vi "deposit.vi"(1 "Elements+Rates":cluster{"Elements":u16[], "Rates":sgl[]}, 2 "# of units":i32, 3 "Input array":T2(array[cluster])) -> (0 "Deposit again?":bool)   [LabVIEW 2012]
uses:
  elements.gbl
  active_process.gbl
  shutter_timeout.gbl
  number_of_sources.gbl
panel:
  in  "Rates":T1
  out "Repeating unit #":i32
  out "Display":string
  in  "Emergency":bool
  in  "Abort":bool
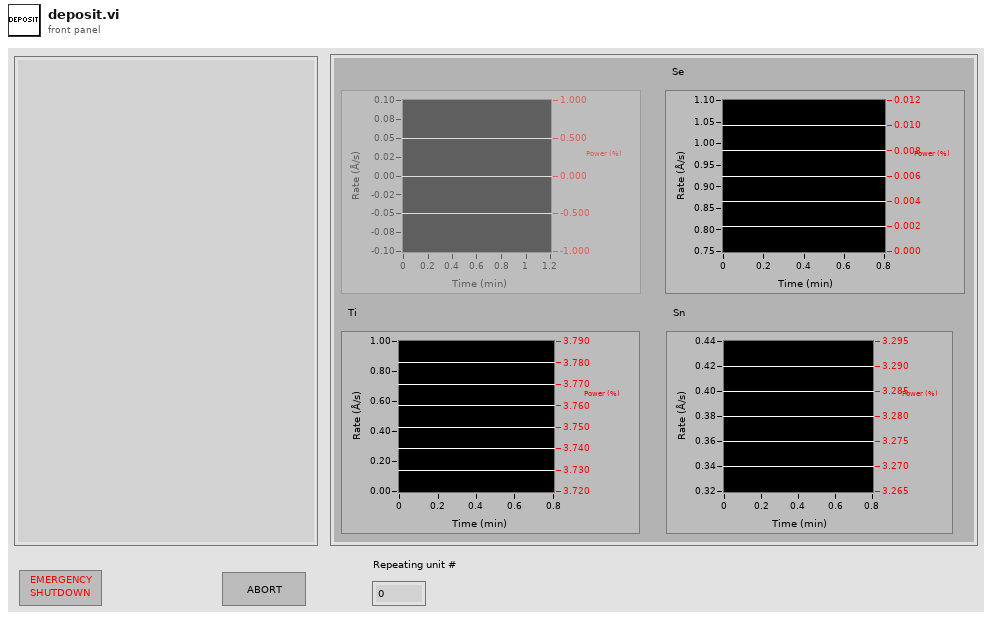
[diagram p1: front panel]
types:
  T1 = cluster{"Rate graph":cluster{cluster{sgl, "Numeric":sgl}[]}[], "Rate graph 2":cluster{cluster{sgl, "Numeric":sgl}[]}[], "Rate graph 3":cluster{cluster{sgl, "Numeric":sgl}[]}[], "Rate graph 4":cluster{cluster{sgl, "Numeric":sgl}[]}[]}
  T2 = cluster{"Elements":u8[][], "T|D":bool[], "T (Å) / D (s)":sgl[], "Repeats":i32}[]
  T3 = enum8{"Enabled", "Disabled", "Disabled and Grayed Out"}
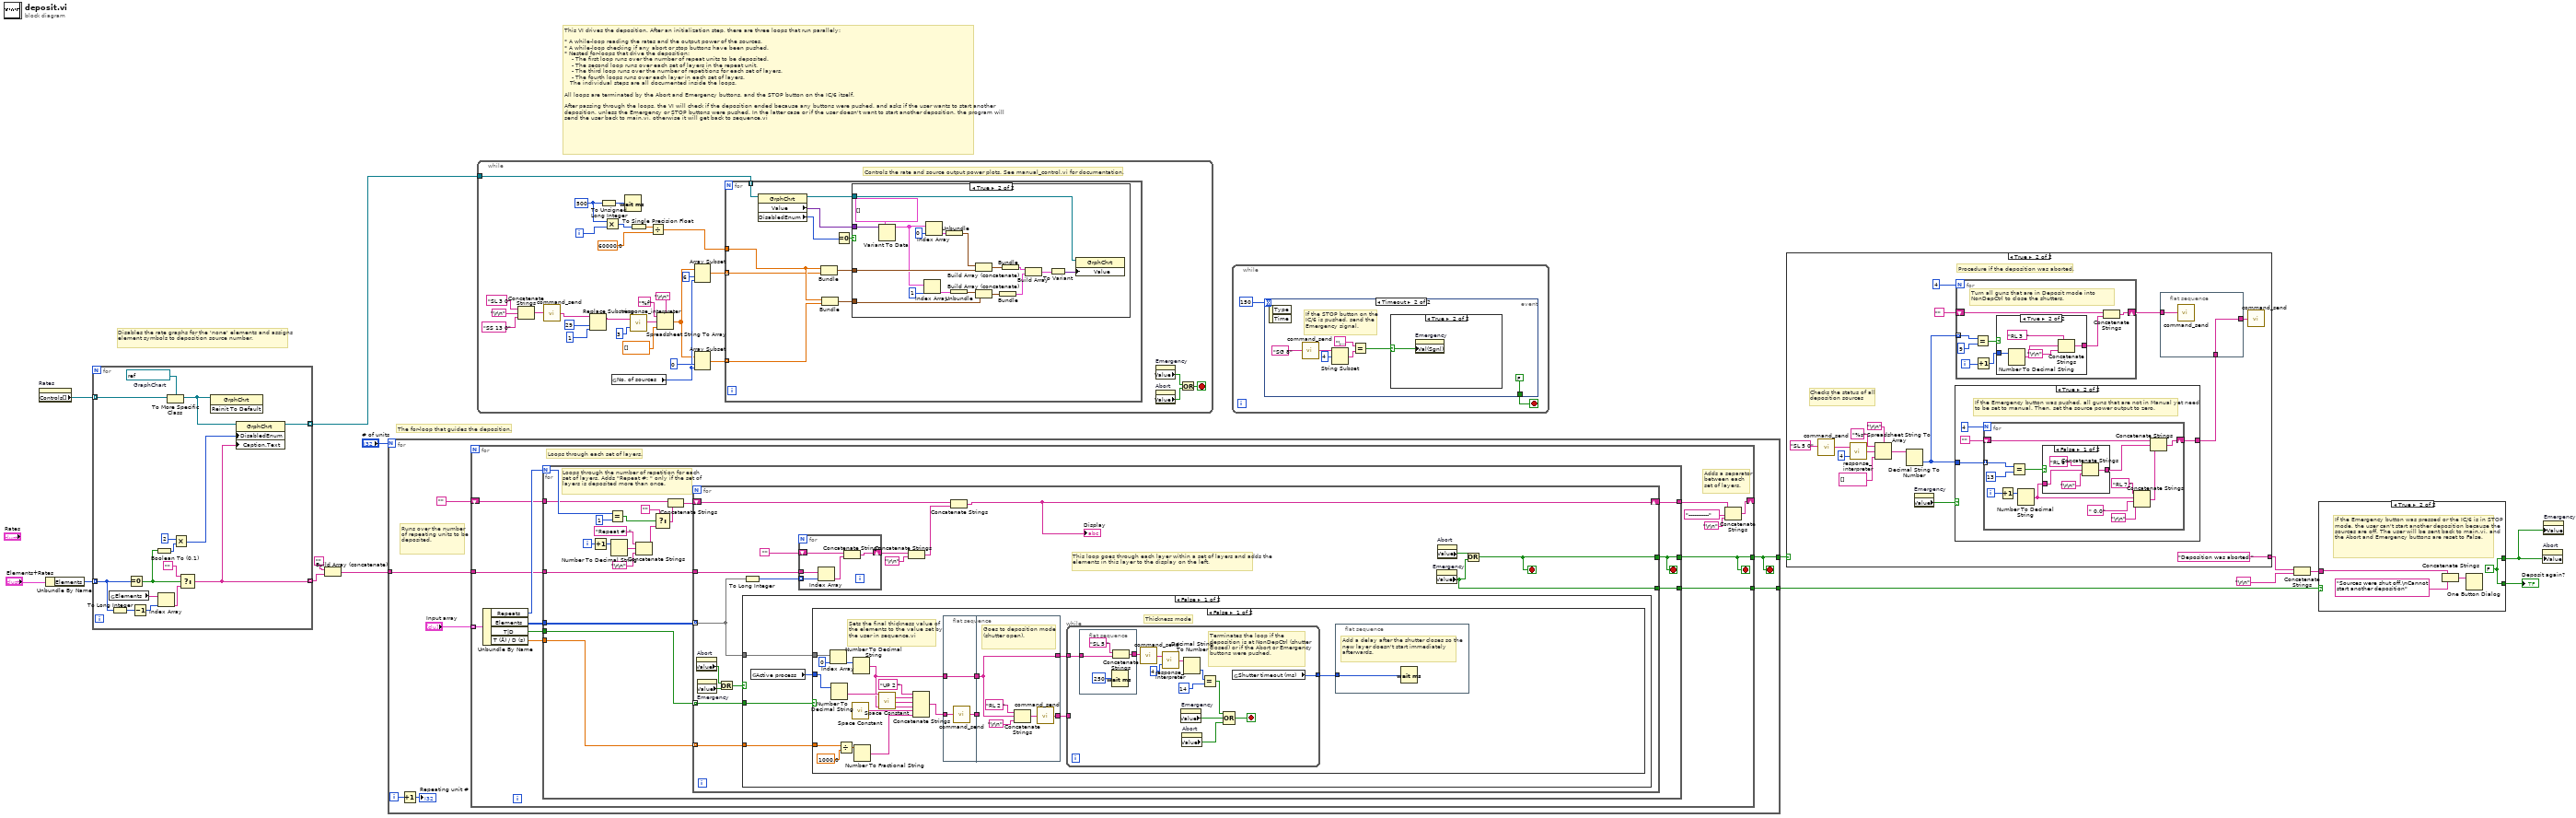
[diagram p0: block diagram]
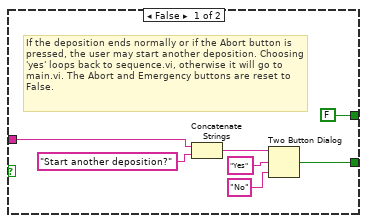
[diagram p2: hidden frame]
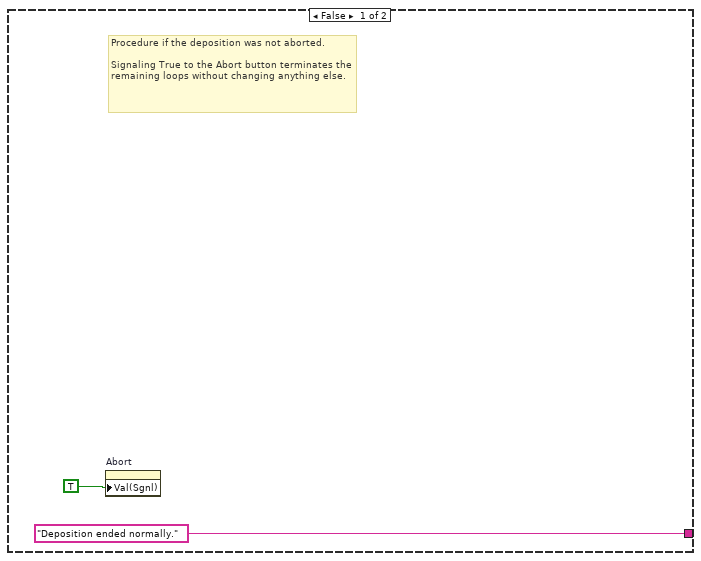
[diagram p3: hidden frame]
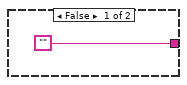
[diagram p4: hidden frame]
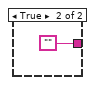
[diagram p5: hidden frame]
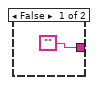
[diagram p6: hidden frame]
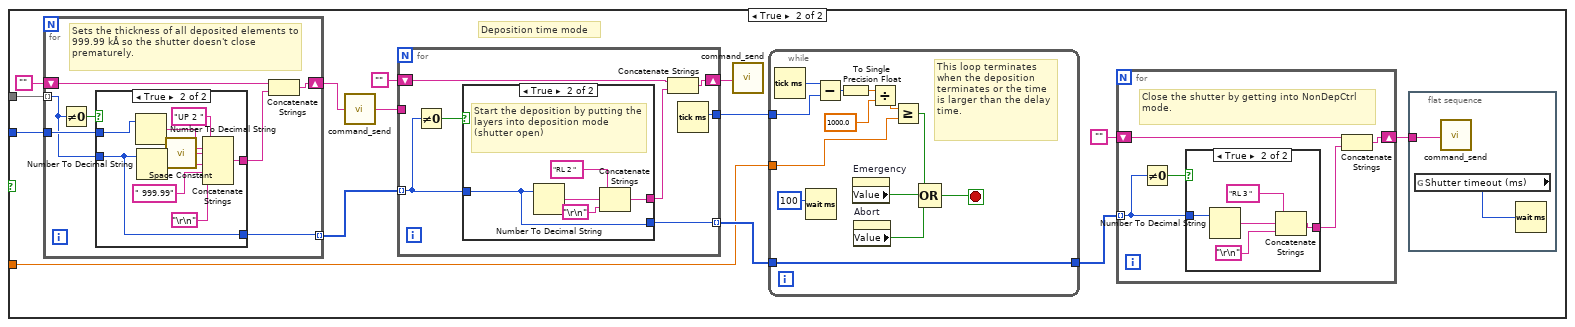
[diagram p7: hidden frame]
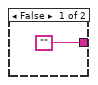
[diagram p8: hidden frame]
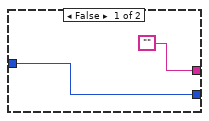
[diagram p9: hidden frame]
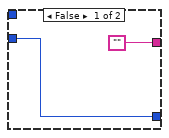
[diagram p10: hidden frame]
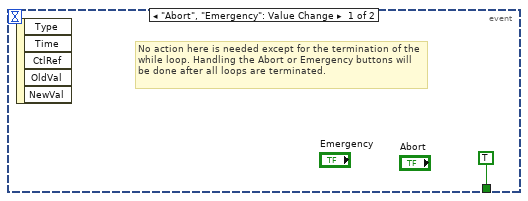
[diagram p13: hidden frame]
diagram:
  # "The for-loop that guides the deposition."
  # "Disables the rate graphs for the 'none' elements and assigns element symbols to deposition source number."
  # "This VI drives the deposition. After an initialization step, there are three loops that run parallely:\n\n* A while-loop reading the rates and the output power of the sources.\n* A while-loop checking if any abort or stop buttons have been pushed. \n* Nested for-loops that drive the deposition:\n    - The first loop runs over the number of repeat units to be deposited.\n    - The second loop runs over each set of layers in the repeat unit.\n    - The third loop runs over the number of repetitions for each set of layers.\n    - The fourth loops runs over each layer in each set of layers.\n   The individual steps are all documented inside the loops.\n\nAll loops are terminated by the Abort and Emergency buttons, and the STOP button on the IC/6 itself.\n\nAfter passing through the loops, the VI will check if the deposition ended because any buttons were pushed, and asks if the user wants to start another deposition, unless the Emergency or STOP buttons were pushed. In the latter case or if the user doesn't want to start another deposition, the program will send the user back to main.vi, otherwise it will get back to sequence.vi"
  n1 = property on="Rates" class="Clust (strict)"() -> ("Controls[]"=w2:refnum<vi>[])  [unwired: 2 in, 2 out]
  n2 = Unbundle By Name("Elements+Rates") -> ("Elements"=w14:u16[])
  n3 = for {
    tunnel: w14 -> [w26] mode=indexing
    tunnel: [w19] -> w8 mode=indexing
    tunnel: w2 -> [w21] mode=indexing
    tunnel: [w17] -> w1 mode=indexing
    w22 = refnum<vi> refnum  # GraphChart
    n4 = global read "elements.gbl" "Elements"() -> (w30:string[])
    n5 = To Long Integer(number=w26) -> (32bit integer=w16:i32)
    n6 = Equal To 0?(x=w26) -> (x = 0?=w23:bool)
    n7 = Decrement(x=w16) -> (x-1=w29:i32)
    n8 = Boolean To (0,1)(Boolean=w23) -> (0, 1=w27:i16)
    n9 = Index Array(array=w30, index=w29) -> (element=w25:string)
    n10 = To More Specific Class(target class=w22, reference=w21) -> (specific class reference=w20:refnum<vi>)  [unwired: 1 in, 1 out]
    n11 = Multiply(x=i16 2, y=w27) -> (x*y=w18:i16)
    n12 = Select(t="", s=w23, f=w25) -> (s? t:f=w19:string)
    n13 = invoke class="GrphChrt" method="Reinit To Default"(reference=w20) -> ()  [unwired: 2 in, 3 out]
    n14 = property class="GrphChrt"(reference=w20, "DisabledEnum"=w18, "Caption.Text"=w19) -> (reference out=w17:refnum<vi>)  [unwired: 1 in, 1 out]
  }
  n15 = Build Array (concatenate)("", w8) -> (w5:string[])
  n16 = for {
    N: "# of units" -> [_]
    tunnel: w5 -> [w34]
    tunnel: [w33] -> w9
    tunnel: [w32] -> w6
    i -> [w36]
    stop <- w33 stop-if-true
    # "Runs over the number of repeating units to be deposited."
    n17 = Increment(x=w36) -> (x+1=→"Repeating unit #":i32)
    n18 = for {
      tunnel: w34 -> [w41]
      shift-right: [w47] -> _
      shift-left: "" -> [w40]
      tunnel: [w46] -> w33
      tunnel: [w45] -> w32
      tunnel: "Input array" -> [w44] mode=indexing
      stop <- w46 stop-if-true
      # "Loops through each set of layers."
      # "Adds a separator between each set of layers."
      n19 = Unbundle By Name(w44) -> ("Repeats"=w43:i32, "Elements"=w42:u8[][], "T|D"=w39:bool[], "T (Å) / D (s)"=w38:sgl[])
      n20 = for {
        N: w43 -> [w57]
        tunnel: w40 -> [w54]
        tunnel: w41 -> [w70]
        tunnel: [w69] -> w48
        tunnel: [w56] -> w46
        tunnel: [w55] -> w45
        tunnel: w42 -> [w53]
        tunnel: w39 -> [w52]
        tunnel: w38 -> [w51]
        i -> [w63]
        stop <- w56 stop-if-true
        # "Loops through the number of repetition for each set of layers. Adds \"Repeat #: \" only if the set of layers is deposited more than once."
        n21 = Increment(x=w63) -> (x+1=w67:i32)
        n22 = Equal?(x=w57, y=1) -> (x = y?=w59:bool)
        n23 = Number To Decimal String(number=w67) -> (decimal integer string=w66:string)  [unwired: 1 in]
        n24 = Concatenate Strings("Repeat #: ", w66, "\r\n") -> (w62:string)
        n25 = Select(t="", s=w59, f=w62) -> (s? t:f=w61:string)
        n26 = Concatenate Strings(w54, w61) -> (w68:string)
        n27 = for {
          tunnel: w53 -> [w85] mode=indexing
          tunnel: w52 -> [w87] mode=indexing
          tunnel: w51 -> [w86] mode=indexing
          shift-right: [w78] -> w69
          shift-left: w68 -> [w80]
          tunnel: w70 -> [w84]
          tunnel: [w75] -> w56
          tunnel: [w76] -> w55
          stop <- w75 stop-if-true
          # "This loop goes through each layer within a set of layers and adds the elements in this layer to the display on the left."
          n28 = property on="Abort" class="Bool (strict)"() -> ("Value"=w72:bool)  [unwired: 2 in, 2 out]
          n29 = property on="Emergency" class="Bool (strict)"() -> ("Value"=w73:bool)  [unwired: 2 in, 2 out]
          n30 = Or(x=w72, y=w73) -> (x .or. y?=w74:bool)
          n31 = case shown="False" w74 {
            tunnel: w87 -> [w91 _]
            tunnel: w86 -> [w90 _]
            tunnel: w85 -> [w89 _]
            frame False {
              n32 = global read "active_process.gbl" "Active process"() -> (w88:i32)
              n33 = case shown="False" w91 {
                tunnel: w90 -> [w107 w141]
                tunnel: w89 -> [w98 w149]
                tunnel: w88 -> [w92 w136]
                frame False {
                  # "Sets the final thickness value of the elements to the value set by the user in sequence.vi"
                  # "Thickness mode"
                  n34 = Index Array(array=w98, index=0) -> (element=w109:u8)
                  n35 = Number To Decimal String(number=w92) -> (decimal integer string=w94:string)  [unwired: 1 in]
                  n36 = Divide(x=w107, y=sgl 1000.0) -> (x/y=w105:sgl)
                  n37 = call <vilib>:"Space Constant.vi"() -> ("String"=w108:string)
                  n38 = Number To Decimal String(number=w109) -> (decimal integer string=w93:string)  [unwired: 1 in]
                  n39 = Number To Fractional String(number=w105) -> (F-format string=w104:string)  [unwired: 3 in]
                  n40 = call <vilib>:"Space Constant.vi"() -> ("String"=w95:string)
                  n41 = Concatenate Strings("UP 2 ", w94, w95, w93, w108, w104) -> (w103:string)
                  n42 = flat-sequence {
                    tunnel: w103 -> [w130]
                    tunnel: w93 -> [w129]
                    tunnel: [w129] -> w102
                    tunnel: [w128] -> w97
                    tunnel: w102 -> [w132]
                    tunnel: [w132] -> w100
                    tunnel: [w131] -> w99
                    tunnel: w97 -> [_]
                    frame #0 {
                      n43 = call "command_send.vi"("Commands"=w130) -> ("Response"=w128:string)
                    }
                    frame #1 {
                      # "Goes to deposition mode (shutter open)."
                      n44 = Concatenate Strings("RL 2 ", w132, "\r\n") -> (w133:string)
                      n45 = call "command_send.vi"("Commands"=w133) -> ("Response"=w131:string)
                    }
                  }
                  n46 = while {
                    tunnel: [w111] -> w101
                    tunnel: w100 -> [w112]
                    tunnel: w99 -> [_]
                    stop <- w113 stop-if-true
                    # "Terminates the loop if the deposition is at NonDepCtrl (shutter closed) or if the Abort or Emergency buttons were pushed."
                    n47 = flat-sequence {
                      tunnel: [w125] -> w120
                      tunnel: w112 -> [w124]
                      frame #0 {
                        n48 = Wait (ms)(milliseconds to wait=u32 250) -> ()  [unwired: 1 out]
                        n49 = Concatenate Strings("SL 5 ", w124) -> (w125:string)
                      }
                    }
                    n50 = call "command_send.vi"("Commands"=w120) -> ("Response"=w119:string)
                    n51 = call "response_interpreter.vi"("Response type"=u16 4, "Response hex"=w119) -> ("Response (readable)"=w116:string)
                    n52 = property on="Emergency" class="Bool (strict)"() -> ("Value"=w121:bool)  [unwired: 2 in, 2 out]
                    n53 = property on="Abort" class="Bool (strict)"() -> ("Value"=w122:bool)  [unwired: 2 in, 2 out]
                    n54 = Decimal String To Number(string=w116) -> (number=w115:i32)  [unwired: 2 in, 1 out]
                    n55 = Equal?(x=w115, y=14) -> (x = y?=w114:bool)
                    n56 = Compound Arithmetic op=OR(w114, w121, w122) -> (w113:bool)
                    n57 = global read "shutter_timeout.gbl" "Shutter timeout (ms)"() -> (w111:u32)
                  }
                  n58 = flat-sequence {
                    tunnel: w101 -> [w127]
                    frame #0 {
                      # "Add a delay after the shutter closes so the new layer doesn't start immediately afterwards."
                      n59 = Wait (ms)(milliseconds to wait=w127) -> ()  [unwired: 1 out]
                    }
                  }
                }
                frame True {
                  # "Deposition time mode"
                  n60 = for {
                    tunnel: w149 -> [w190] mode=indexing
                    shift-right: [w193] -> w147
                    shift-left: "" -> [w195]
                    tunnel: [w192] -> w146 mode=indexing
                    tunnel: w136 -> [w191]
                    # "Sets the thickness of all deposited elements to 999.99 kÅ so the shutter doesn't close prematurely."
                    n61 = Not Equal To 0?(x=w190) -> (x != 0?=w196:bool)
                    n62 = case shown="True" w196 {
                      tunnel: w190 -> [w197 w203]
                      tunnel: ["" w204] -> w194
                      tunnel: [w197 w203] -> w192
                      tunnel: w191 -> [_ w199]
                      frame False {
                      }
                      frame True {
                        n63 = Number To Decimal String(number=w199) -> (decimal integer string=w200:string)  [unwired: 1 in]
                        n64 = Number To Decimal String(number=w203) -> (decimal integer string=w206:string)  [unwired: 1 in]
                        n65 = call <vilib>:"Space Constant.vi"() -> ("String"=w202:string)
                        n66 = Concatenate Strings("UP 2 ", w200, w202, w206, " 999.99", "\r\n") -> (w204:string)
                      }
                    }
                    n67 = Concatenate Strings(w195, w194) -> (w193:string)
                  }
                  n68 = call "command_send.vi"("Commands"=w147) -> ("Response"=w137:string)
                  n69 = for {
                    tunnel: w146 -> [w181] mode=indexing
                    shift-right: [w178] -> w144
                    shift-left: "" -> [w180]
                    tunnel: [w177] -> w142 mode=indexing
                    tunnel: [w176] -> w143
                    tunnel: w137 -> [_]
                    n70 = Not Equal To 0?(x=w181) -> (x != 0?=w182:bool)
                    n71 = case shown="True" w182 {
                      tunnel: w181 -> [w183 w186]
                      tunnel: ["" w187] -> w179
                      tunnel: [w183 w186] -> w177
                      frame False {
                      }
                      frame True {
                        # "Start the deposition by putting the layers into deposition mode (shutter open)"
                        n72 = Number To Decimal String(number=w186) -> (decimal integer string=w189:string)  [unwired: 1 in]
                        n73 = Concatenate Strings("RL 2 ", w189, "\r\n") -> (w187:string)
                      }
                    }
                    n74 = Concatenate Strings(w180, w179) -> (w178:string)
                    n75 = Tick Count (ms)() -> (millisecond timer value=w176:u32)
                  }
                  n76 = call "command_send.vi"("Commands"=w144) -> ()  [unwired: 1 out]
                  n77 = while {
                    tunnel: w143 -> [w174]
                    tunnel: w141 -> [w170]
                    tunnel: w142 -> [w164]
                    tunnel: [w164] -> w138
                    stop <- w165 stop-if-true
                    # "This loop terminates when the deposition terminates or the time is larger than the delay time."
                    n78 = Tick Count (ms)() -> (millisecond timer value=w175:u32)
                    n79 = Wait (ms)(milliseconds to wait=u32 100) -> ()  [unwired: 1 out]
                    n80 = Subtract(x=w175, y=w174) -> (x-y=w173:u32)
                    n81 = To Single Precision Float(number=w173) -> (single precision float=w163:sgl)
                    n82 = property on="Emergency" class="Bool (strict)"() -> ("Value"=w167:bool)  [unwired: 2 in, 2 out]
                    n83 = property on="Abort" class="Bool (strict)"() -> ("Value"=w168:bool)  [unwired: 2 in, 2 out]
                    n84 = Divide(x=w163, y=sgl 1000.0) -> (x/y=w171:sgl)
                    n85 = Greater Or Equal?(x=w171, y=w170) -> (x >= y?=w166:bool)
                    n86 = Compound Arithmetic op=OR(w166, w167, w168) -> (w165:bool)
                  }
                  n87 = for {
                    tunnel: w138 -> [w155] mode=indexing
                    shift-right: [w152] -> w140
                    shift-left: "" -> [w154]
                    # "Close the shutter by getting into NonDepCtrl mode."
                    n88 = Not Equal To 0?(x=w155) -> (x != 0?=w156:bool)
                    n89 = case shown="True" w156 {
                      tunnel: w155 -> [_ w159]
                      tunnel: ["" w160] -> w153
                      frame False {
                      }
                      frame True {
                        n90 = Number To Decimal String(number=w159) -> (decimal integer string=w162:string)  [unwired: 1 in]
                        n91 = Concatenate Strings("RL 3 ", w162, "\r\n") -> (w160:string)
                      }
                    }
                    n92 = Concatenate Strings(w154, w153) -> (w152:string)
                  }
                  n93 = flat-sequence {
                    tunnel: w140 -> [w151]
                    frame #0 {
                      n94 = global read "shutter_timeout.gbl" "Shutter timeout (ms)"() -> (w150:u32)
                      n95 = call "command_send.vi"("Commands"=w151) -> ()  [unwired: 1 out]
                      n96 = Wait (ms)(milliseconds to wait=w150) -> ()  [unwired: 1 out]
                    }
                  }
                }
              }
            }
            frame True {
              # "If this condition isn't set, the VI will start depositing the current layer even when it should abort the deposition."
            }
          }
          n97 = To Long Integer(number=w85) -> (32bit integer=w71:i32[])
          n98 = for {
            tunnel: w71 -> [w208] mode=indexing
            tunnel: w84 -> [w209]
            shift-right: [w211] -> w82
            shift-left: "" -> [w212]
            n99 = Index Array(array=w209, index=w208) -> (element=w210:string)
            n100 = Concatenate Strings(w212, w210) -> (w211:string)
          }
          n101 = Concatenate Strings(w82, "\r\n") -> (w79:string)
          n102 = Concatenate Strings(w80, w79) -> (w78:string)
          "Display" <- w78
          n103 = property on="Emergency" class="Bool (strict)"() -> ("Value"=w76:bool)  [unwired: 2 in, 2 out]
          n104 = property on="Abort" class="Bool (strict)"() -> ("Value"=w77:bool)  [unwired: 2 in, 2 out]
          n105 = Or(x=w77, y=w76) -> (x .or. y?=w75:bool)
        }
      }
      n106 = Concatenate Strings(w48, "-----------", "\r\n") -> (w47:string)
    }
  }
  n107 = while {
    tunnel: w1 -> [w234]
    i -> [w239]
    stop <- w240 stop-if-true
    w238 = 500
    # "Controls the rate and source output power plots. See manual_control.vi for documentation."
    n108 = Concatenate Strings("SL 3 0", "\r\n", "SS 13 0") -> (w225:string)
    n109 = call "command_send.vi"("Commands"=w225) -> ("Response"=w216:string)
    n110 = Replace Substring(2:1, 3:29, 5:w216) -> (1:w217:string)  [unwired: 1 in, 1 out]
    n111 = To Unsigned Long Integer(number=w238) -> (unsigned 32bit integer=w213:u32)
    n112 = Multiply(x=w238, y=w239) -> (x*y=w237:i32)
    n113 = global read "number_of_sources.gbl" "No. of sources"() -> (w220:i32)
    n114 = Wait (ms)(milliseconds to wait=w213) -> ()  [unwired: 1 out]
    n115 = call "response_interpreter.vi"("Response type"=u16 3, "Response hex"=w217) -> ("Response (readable)"=w230:string)
    n116 = To Single Precision Float(number=w237) -> (single precision float=w218:sgl)
    n117 = Divide(x=w218, y=sgl 60000.0) -> (x/y=w235:sgl)
    n118 = Spreadsheet String To Array(delimiter (Tab)="\r\n", format string="%f", spreadsheet string=w230, array type (2D Dbl)=sgl[] []) -> (array=w219:sgl[])
    n119 = Array Subset(array=w219, index=6, length=w220) -> (w224:sgl[])
    n120 = Array Subset(array=w219, index=0, length=w220) -> (w223:sgl[])
    n121 = for {
      tunnel: w224 -> [w248] mode=indexing
      tunnel: w235 -> [w252]
      tunnel: w223 -> [w247] mode=indexing
      tunnel: w234 -> [w246] mode=indexing
      n122 = property class="GrphChrt"(reference=w246) -> (reference out=w245:refnum<vi>, "Value"=w243:variant, "DisabledEnum"=w244:T3)  [unwired: 1 in, 1 out]
      n123 = Bundle(w252, w248) -> (w250:cluster{sgl, sgl})  [unwired: 1 in]
      n124 = Bundle(w252, w247) -> (w251:cluster{sgl, sgl})  [unwired: 1 in]
      n125 = Equal To 0?(x=w244) -> (x = 0?=w249:bool)
      n126 = case shown="True" w249 {
        tunnel: w251 -> [_ w266]
        tunnel: w250 -> [_ w262]
        tunnel: w243 -> [_ w254]
        tunnel: w245 -> [_ w257]
        frame False {
        }
        frame True {
          n127 = Variant To Data(type=cluster{cluster{sgl, sgl}[]}[] [], Variant=w254) -> (data=w255:cluster{cluster{sgl, sgl}[]}[])  [unwired: 1 in, 1 out]
          n128 = Index Array(array=w255, index=1) -> (element=w260:cluster{cluster{sgl, sgl}[]})
          n129 = Index Array(array=w255, index=0) -> (element=w263:cluster{cluster{sgl, sgl}[]})
          n130 = Unbundle(w263) -> (w261:cluster{sgl, sgl}[])
          n131 = Unbundle(w260) -> (w259:cluster{sgl, sgl}[])
          n132 = Build Array (concatenate)(w261, w262) -> (w269:cluster{sgl, sgl}[])
          n133 = Build Array (concatenate)(w259, w266) -> (w270:cluster{sgl, sgl}[])
          n134 = Bundle(w270) -> (w267:cluster{cluster{sgl, sgl}[]})  [unwired: 1 in]
          n135 = Bundle(w269) -> (w268:cluster{cluster{sgl, sgl}[]})  [unwired: 1 in]
          n136 = Build Array(w268, w267) -> (w258:cluster{cluster{sgl, sgl}[]}[])
          n137 = To Variant(anything=w258) -> (Variant=w256:variant)
          n138 = property class="GrphChrt"(reference=w257, "Value"=w256) -> ()  [unwired: 1 in, 2 out]
        }
      }
    }
    n139 = property on="Emergency" class="Bool (strict)"() -> ("Value"=w242:bool)  [unwired: 2 in, 2 out]
    n140 = property on="Abort" class="Bool (strict)"() -> ("Value"=w241:bool)  [unwired: 2 in, 2 out]
    n141 = Or(x=w242, y=w241) -> (x .or. y?=w240:bool)
  }
  n142 = while {
    stop <- w272 stop-if-true
    n143 = event shown="[1] Timeout" {
      selector: _ -> [_ _]
      dyn-events: _ -> [_ _]
      timeout: 150 -> [_ _]
      tunnel: [TRUE FALSE] -> w272
      event "Abort", "Emergency": Value Change {
        # "No action here is needed except for the termination of the while loop. Handling the Abort or Emergency buttons will be done after all loops are terminated."
        n144 = event-data() -> ()  [unwired: 1 in, 5 out]
      }
      event Timeout {
        # "If the STOP button on the IC/6 is pushed, send the Emergency signal."
        n145 = event-data() -> ()  [unwired: 1 in, 2 out]
        n146 = call "command_send.vi"("Commands"="SG 8") -> ("Response"=w279:string)
        n147 = String Subset(string=w279, offset (0)=4) -> (substring=w276:string)  [unwired: 1 in]
        n148 = Equal?(x="\u0006", y=w276) -> (x = y?=w274:bool)
        n149 = case shown="True" w274 {
          selector: w274 -> [_ w281]
          frame False {
          }
          frame True {
            n150 = property on="Emergency" class="Bool (strict)"("Val(Sgnl)"=w281) -> ()  [unwired: 2 in, 2 out]
          }
        }
      }
    }
  }
  n151 = case shown="True" w9 {
    tunnel: ["Deposition ended normally." "Deposition was aborted."] -> w3
    frame False {
      # "Procedure if the deposition was not aborted.\n\nSignaling True to the Abort button terminates the remaining loops without changing anything else."
      n152 = property on="Abort" class="Bool (strict)"("Val(Sgnl)"=TRUE) -> ()  [unwired: 2 in, 2 out]
    }
    frame True {
      # "Procedure if the deposition was aborted."
      # "Checks the status of all deposition sources"
      n153 = call "command_send.vi"("Commands"="SL 5 0") -> ("Response"=w291:string)
      n154 = call "response_interpreter.vi"("Response type"=u16 4, "Response hex"=w291) -> ("Response (readable)"=w294:string)
      n155 = Spreadsheet String To Array(delimiter (Tab)="\r\n", format string="%s", spreadsheet string=w294, array type (2D Dbl)=string[] []) -> (array=w293:string[])
      n156 = Decimal String To Number(string=w293) -> (number=w292:i32[])  [unwired: 2 in, 1 out]
      n157 = property on="Emergency" class="Bool (strict)"() -> ("Value"=w288:bool)  [unwired: 2 in, 2 out]
      n158 = case shown="True" w288 {
        tunnel: ["" w306] -> w285
        tunnel: w292 -> [_ w305]
        frame False {
        }
        frame True {
          # "If the Emergency button was pushed, all guns that are not in Manual yet need to be set to manual. Then, set the source power output to zero."
          n159 = for {
            N: 4 -> [_]
            shift-right: [w317] -> w306
            shift-left: "" -> [w318]
            tunnel: w305 -> [w315] mode=indexing
            i -> [w319]
            n160 = Increment(x=w319) -> (x+1=w313:i32)
            n161 = Equal?(x=w315, y=13) -> (x = y?=w316:bool)
            n162 = Number To Decimal String(number=w313) -> (decimal integer string=w308:string)  [unwired: 1 in]
            n163 = case shown="False" w316 {
              tunnel: w308 -> [w322 _]
              tunnel: [w320 ""] -> w312
              frame False {
                n164 = Concatenate Strings("RL 6 ", w322, "\r\n") -> (w320:string)
              }
              frame True {
              }
            }
            n165 = Concatenate Strings("RL 7 ", w308, " 0.0", "\r\n") -> (w307:string)
            n166 = Concatenate Strings(w318, w312, w307) -> (w317:string)
          }
        }
      }
      n167 = for {
        N: 4 -> [_]
        tunnel: w292 -> [w332] mode=indexing
        shift-right: [w330] -> w284
        shift-left: "" -> [w329]
        i -> [w327]
        # "Turn all guns that are in Deposit mode into NonDepCtrl to close the shutters."
        n168 = Equal?(x=w332, y=9) -> (x = y?=w328:bool)
        n169 = Increment(x=w327) -> (x+1=w326:i32)
        n170 = case shown="True" w328 {
          tunnel: w326 -> [_ w338]
          tunnel: ["" w336] -> w325
          frame False {
          }
          frame True {
            n171 = Number To Decimal String(number=w338) -> (decimal integer string=w337:string)  [unwired: 1 in]
            n172 = Concatenate Strings("RL 3  ", w337, "\r\n") -> (w336:string)
          }
        }
        n173 = Concatenate Strings(w329, w325) -> (w330:string)
      }
      n174 = flat-sequence {
        tunnel: [w301] -> w286
        tunnel: w285 -> [w301]
        tunnel: w284 -> [w300]
        frame #0 {
          n175 = call "command_send.vi"("Commands"=w300) -> ()  [unwired: 1 out]
        }
      }
      n176 = call "command_send.vi"("Commands"=w286) -> ()  [unwired: 1 out]
    }
  }
  n177 = Concatenate Strings(w3, "\r\n") -> (w12:string)
  n178 = case shown="True" w6 {
    tunnel: w12 -> [w344 w348]
    tunnel: [w340 w346] -> w11
    tunnel: [FALSE w346] -> w10
    frame False {
      # "If the deposition ends normally or if the Abort button is pressed, the user may start another deposition. Choosing 'yes' loops back to sequence.vi, otherwise it will go to main.vi. The Abort and Emergency buttons are reset to False."
      n179 = Concatenate Strings(w344, "Start another deposition?") -> (w343:string)
      n180 = Two Button Dialog(message=w343, 1:"No", 2:"Yes") -> (T button?=w340:bool)
    }
    frame True {
      w346 = FALSE
      # "If the Emergency button was pressed or the IC/6 is in STOP mode, the user can't start another deposition because the sources are off. The user will be sent back to main.vi, and the Abort and Emergency buttons are reset to False."
      n181 = Concatenate Strings(w348, "Sources were shut off.\nCannot start another deposition") -> (w347:string)
      n182 = One Button Dialog(message=w347) -> ()  [unwired: 1 in, 1 out]
    }
  }
  "Deposit again?" <- w11
  n183 = property on="Abort" class="Bool (strict)"("Value"=w10) -> ()  [unwired: 2 in, 2 out]
  n184 = property on="Emergency" class="Bool (strict)"("Value"=w10) -> ()  [unwired: 2 in, 2 out]
